vi "AE_Continuous.vi"() -> ()   [LabVIEW 2012]
uses:
  <vilib>/DAQmx/read.llb/DAQmx Read (Analog 1D Wfm NChan NSamp).vi
  <vilib>/DAQmx/create/channels.llb/DAQmx Create Channel (AI-Voltage-Basic).vi
  <vilib>/DAQmx/configure/timing.llb/DAQmx Timing (Sample Clock).vi
  <vilib>/DAQmx/miscellaneous.llb/DAQmx Fill In Error Info.vi
panel:
  in  "Physical Channel":tag="Dev1/ai7"
  in  "Gain":u16(ring)=1 items=["20 dB", "40 dB", "60 dB"]
  in  "Samples":i32=500 min=0 max=1000
  in  "stop":bool
  in  "Test Name":string="test"
  in  "Storage Directory":path=path "C:/Users/User/Desktop/Users_2013-2014/Michael Rossol"
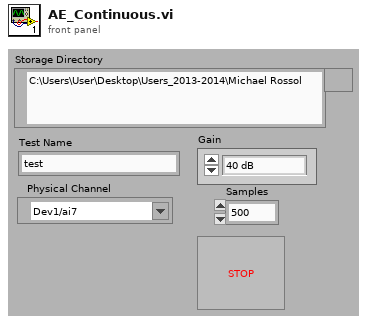
[diagram p1: front panel]
types:
  T1 = enum16{"open", "open or create", "create or replace", "create", "open (read only)"}
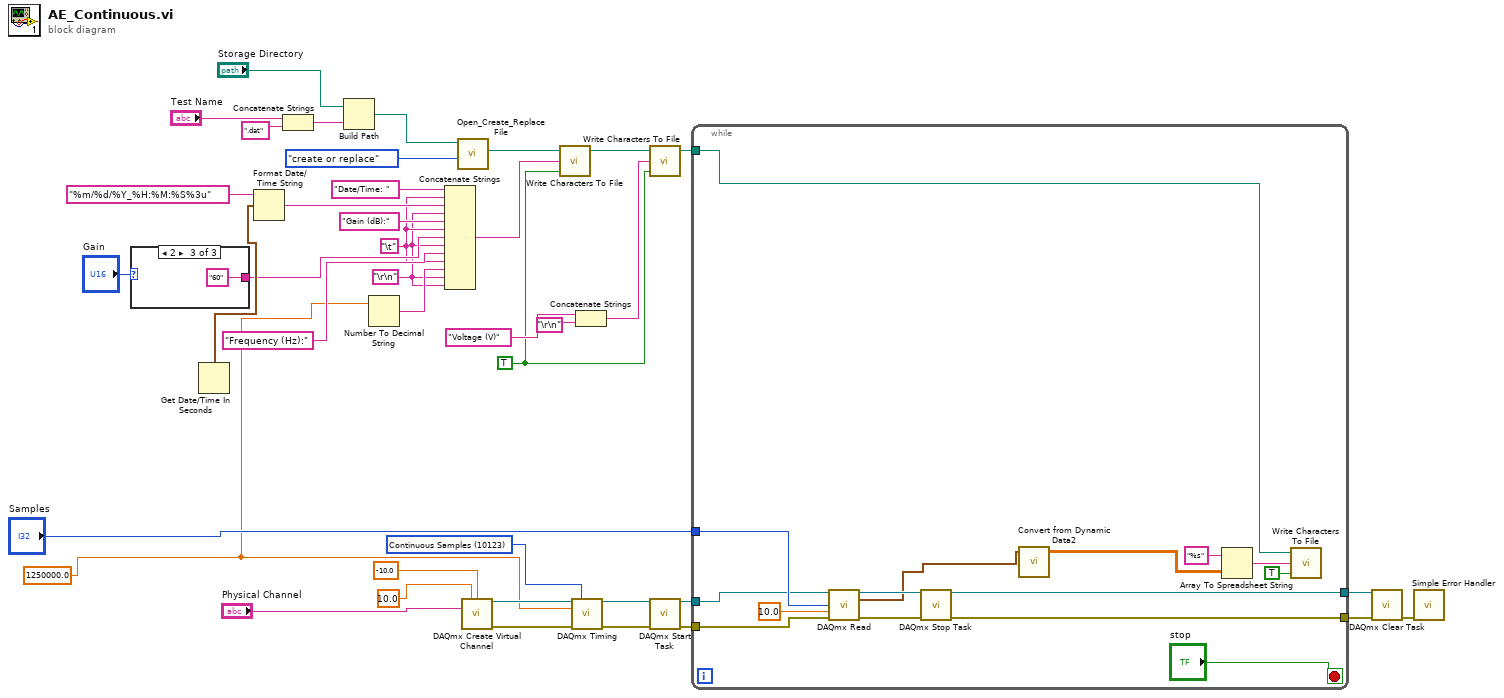
[diagram p0: block diagram]
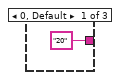
[diagram p2: hidden frame]
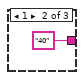
[diagram p3: hidden frame]
diagram:
  w15 = 10123 items=["Finite Samples"=10178, "Continuous Samples"=10123] ("sample mode")
  w1 = 1250000.0 ("x")
  w9 = "\t"
  w7 = "\r\n"
  w26 = TRUE ("append to file? (new file:F)")
  n1 = case shown="2" "Gain" {
    tunnel: ["20" ("string") "40" ("string") "60" ("string")] -> w20
    frame 0, Default {
    }
    frame 1 {
    }
    frame 2 {
    }
  }
  n2 = Get Date/Time In Seconds() -> (seconds since 1Jan1904=w29:timestamp)
  n3 = Format Date/Time String(time format string (%c)="%m/%d/%Y_%H:%M:%S%3u", seconds (now)=w29) -> (date/time string=w30:string)  [unwired: 1 in]
  n4 = Concatenate Strings("Test Name", ".dat" ("string")) -> (w33:string)
  n5 = Build Path(base path="Storage Directory", name or relative path=w33) -> (appended path=w31:path)
  n6 = Number To Decimal String(number=w1) -> (decimal integer string=w8:string)  [unwired: 1 in]
  n7 = Concatenate Strings("Date/Time: ", w9, w30, w7, "Gain (dB):" ("string"), w9, w20, w7, "Frequency (Hz):" ("string"), w9, w8, w7, w7) -> (w40:string)
  n8 = call <vilib>:"Open_Create_Replace File.vi"("function (open:0)"=T1."create or replace", "file path"=w31) -> ("new file path"=w36:path)  [unwired: 6 in, 3 out]
  n9 = call-poly <vilib>:"DAQmx Create Virtual Channel.vi"("maximum value"=10.0, "minimum value"=-10.0, "physical channels"="Physical Channel") -> ("task out"=w17:refnum<k21>, "error out"=w16:errorcluster)  [unwired: 11 in]
  n10 = call <vilib>:"Write Characters To File.vi"("append to file? (new file:F)"=w26, "character string"=w40, "file path (dialog if empty)"=w36) -> ("new file path (Not A Path if cancelled)"=w24:path)  [unwired: 2 in]
  n11 = call-poly <vilib>:"DAQmx Timing.vi"("task/channels in"=w17, "sample mode"=w15, "rate"=w1, "error in"=w16) -> ("task out"=w5:refnum<k21>, "error out"=w6:errorcluster)  [unwired: 10 in]
  n12 = Concatenate Strings("Voltage (V)" ("string"), "\r\n") -> (w25:string)
  n13 = call <vilib>:"Write Characters To File.vi"("append to file? (new file:F)"=w26, "character string"=w25, "file path (dialog if empty)"=w24) -> ("new file path (Not A Path if cancelled)"=w23:path)  [unwired: 2 in]
  n14 = call <vilib>:"DAQmx Start Task.vi"("task/channels in"=w5, "error in"=w6) -> ("task out"=w4:refnum<k21>, "error out"=w3:errorcluster)  [unwired: 12 in]
  n15 = while {
    tunnel: w23 -> [w55]
    tunnel: "Samples" -> [w48]
    tunnel: [w50] -> w13
    tunnel: [w49] -> w12
    tunnel: w4 -> [w47]
    tunnel: w3 -> [w46]
    stop <- "stop" stop-if-true
    n16 = call-poly <vilib>:"DAQmx Read.vi"("task/channels in"=w47, "number of samples per channel"=w48, "timeout"=10.0, "error in"=w46) -> ("task out"=w51:refnum<k21>, "data"=w45:waveform(dbl)[], "error out"=w52:errorcluster)  [unwired: 9 in]
    n17 = call <vilib>:"DAQmx Stop Task.vi"("task/channels in"=w51, "error in"=w52) -> ("task out"=w49:refnum<k21>, "error out"=w50:errorcluster)  [unwired: 12 in]
    n18 = call "Convert from Dynamic Data2"("Dynamic Data Type"=w45) -> ("Array"=w44:dbl[][])  [unwired: 3 in]
    n19 = Array To Spreadsheet String(array=w44, 3:"%s" ("format string")) -> (spreadsheet string=w56:string)  [unwired: 1 in]
    n20 = call <vilib>:"Write Characters To File.vi"("append to file? (new file:F)"=TRUE, "character string"=w56, "file path (dialog if empty)"=w55) -> ()  [unwired: 2 in, 1 out]
  }
  n21 = call <vilib>:"DAQmx Clear Task.vi"("task in"=w12, "error in"=w13) -> ("error out"=w14:errorcluster)  [unwired: 13 in]
  n22 = call <vilib>:"Simple Error Handler.vi"("error in (no error)"=w14) -> ()  [unwired: 4 in, 5 out]
